vi "Zaber A Series Sinusoidal Move.vi"() -> ()   [LabVIEW 2015]
doc: "Demonstrates how the Move Sin VI can be used to easily set-up and run a sinusoidal motion. This example also records the position and displays a position vs time chart during the motion."
uses:
  Zaber A Series.lvlib
panel:
  out "Position Graph":waveform(dbl)(graph)
  in  "stop":bool
  in  "Period in milliseconds":dbl=0.2 min=0.2 step=0.1 format="%#.1f"
  in  "Units (0: microsteps)":u16(ring) items=["microsteps", "microns", "millimeters", "inches", "degrees"]
  in  "Amplitude (half of pk - pk)":dbl
  in  "Device and Axis":string
  in  "Microstep Size (0)":dbl
  in  "VISA resource name":refnum<visa-resource-name>
  # "(c) 2017 Zaber Technologies.  ALL RIGHTS RESERVED."
  # "This example demonstrates the sinusoidal movement commands. \n\nSelect a serial port, device number and axis number, then enter the peak \namplitude and period of the sine wave to run. Press STOP\nto stop moving at the end of the next period."
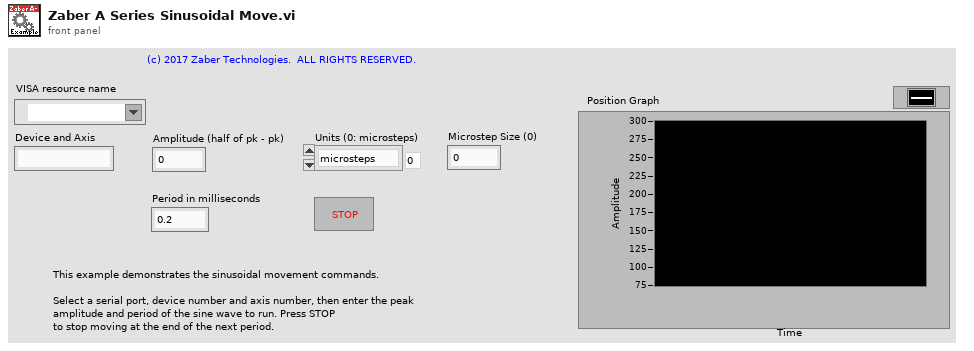
[diagram p1: front panel]
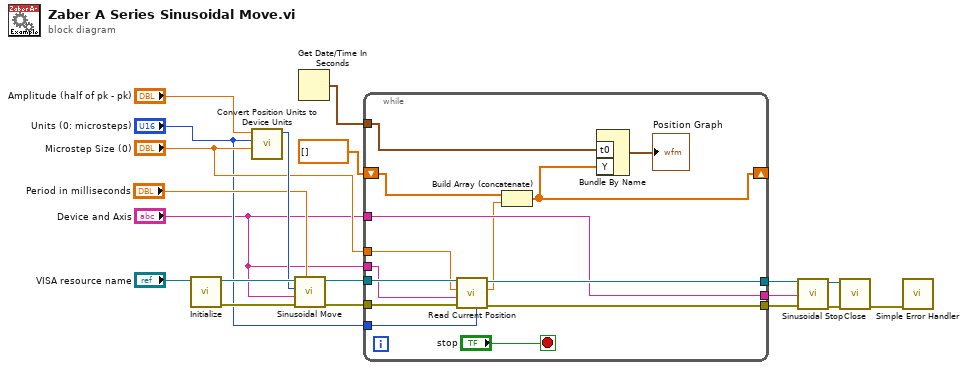
[diagram p0: block diagram]
diagram:
  n1 = call "Initialize.vi"("VISA resource name"="VISA resource name") -> ("error out"=w16:errorcluster, "VISA resource name out"=w17:refnum<visa-resource-name>)  [unwired: 9 in]
  n2 = call "Convert Position Units to Device Units.vi"("Microstep Size (0)"="Microstep Size (0)", "Units (0: microsteps)"="Units (0: microsteps)", "Position (0)"="Amplitude (half of pk - pk)") -> ("Device Position (32-bit)"=w12:i32)  [unwired: 6 in, 2 out]
  n3 = call "Sinusoidal Move.vi"("Period"="Period in milliseconds", "error in (no error)"=w16, "Device and Axis"="Device and Axis", "Amplitude"=w12, "VISA resource name"=w17) -> ("error out"=w8:errorcluster, "VISA resource name out"=w10:refnum<visa-resource-name>)  [unwired: 5 in]
  n4 = Get Date/Time In Seconds() -> (seconds since 1Jan1904=w1:timestamp)
  n5 = while {
    tunnel: w10 -> [w32]
    tunnel: [w31] -> w9
    tunnel: w8 -> [w30]
    tunnel: [w29] -> w7
    tunnel: "Device and Axis" -> [w28]
    tunnel: "Microstep Size (0)" -> [w27]
    tunnel: "Units (0: microsteps)" -> [w26]
    tunnel: "Device and Axis" -> [w25]
    tunnel: [w25] -> w3
    shift-right: [w21] -> _
    shift-left: dbl[] [] -> [w22]
    tunnel: w1 -> [w20]
    stop <- "stop" stop-if-true
    n6 = call "Read Current Position.vi"("Units (0: microsteps)"=w26, "error in (no error)"=w30, "Device and Axis"=w28, "Microstep Size (0)"=w27, "VISA resource name"=w32) -> ("error out"=w29:errorcluster, "Position"=w23:dbl, "VISA resource name out"=w31:refnum<visa-resource-name>)  [unwired: 4 in]
    n7 = Build Array (concatenate)(w22, w23) -> (w21:dbl[])
    n8 = Bundle By Name("t0"=w20, "Y"=w21) -> (→"Position Graph":waveform(dbl))  [unwired: 1 in]
  }
  n9 = call "Sinusoidal Stop.vi"("error in (no error)"=w7, "Device and Axis"=w3, "VISA resource name"=w9) -> ("error out"=w14:errorcluster, "VISA resource name out"=w15:refnum<visa-resource-name>)  [unwired: 7 in]
  n10 = call "Close.vi"("error in (no error)"=w14, "VISA resource name"=w15) -> ("error out"=w18:errorcluster)  [unwired: 9 in]
  n11 = call <vilib>:"Simple Error Handler.vi"("error in (no error)"=w18) -> ()  [unwired: 4 in, 5 out]
